vi "hardware_close_hardware.vi"(8 "error in (no error)":errorcluster, 11 "mcl_piezo in":refnum<class "mcl_piezo.lvclass">) -> (0 "error out":errorcluster, 3 "mcl_piezo out":refnum<class "mcl_piezo.lvclass">)   [LabVIEW 2015, in "mcl_piezo.lvclass"]
uses:
  mcl_piezo.lvclass
  mcl_piezo.lvclass/mcl_piezo.ctl
  Madlib.dll
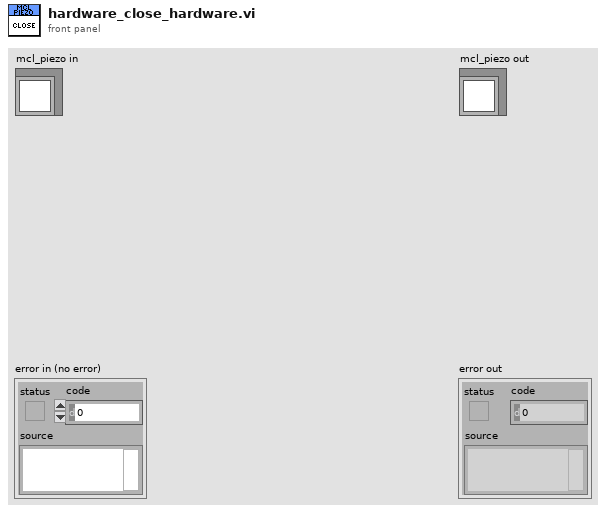
[diagram p1: front panel]
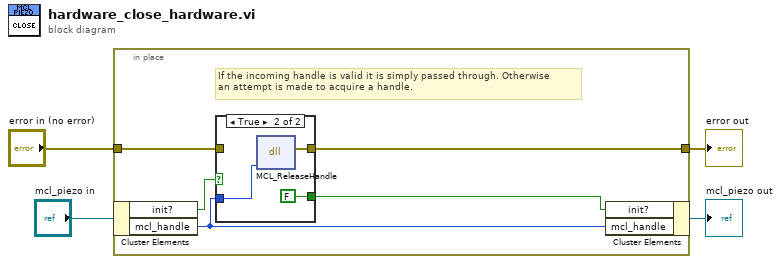
[diagram p0: block diagram]
diagram:
  n1 = in-place {
    in-place-border: "error in (no error)" -> [w9]
    in-place-border: [w8] -> w3
    # "If the incoming handle is valid it is simply passed through. Otherwise\nan attempt is made to acquire a handle."
    n2 = in-place-cluster #1("mcl_piezo in") -> ("init?"=w6:bool, "mcl_handle"=w5:i32)
    n3 = case shown="True" w6 {
      selector: w6 -> [w10 _]
      tunnel: w9 -> [w11 _]
      tunnel: [w11 w12] -> w8
      tunnel: w5 -> [_ w14]
      tunnel: [w10 FALSE] -> w7
      frame False {
      }
      frame True {
        n4 = dll-call lib="C:/Users/MX-Microscope/Documents/LabVIEW Data/lvoop_campus_2018/Stage Class/MCL_3d200/MADLib.dll" fn="MCL_ReleaseHandle"("handle"=w14) -> (error out=w12:errorcluster)  [unwired: 5 in, 1 out]
      }
    }
    n5 = in-place-cluster #1("init?"=w7, "mcl_handle"=w5) -> (→"mcl_piezo out":refnum<class "mcl_piezo.lvclass">)
  }
  "error out" <- w3
